vi "TempVol._activity3.vi"() -> (0 "Volume":dbl(slide) scale=0.0..1000.0, 1 "Temp":dbl(slide) scale=0.0..100.0)   [LabVIEW 2025]
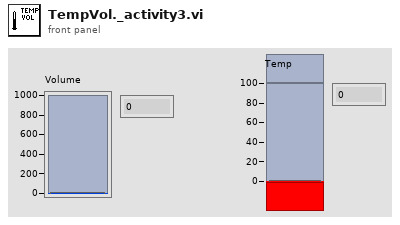
[diagram p1: front panel]
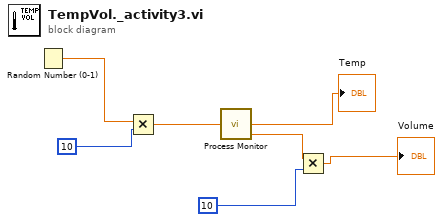
[diagram p0: block diagram]
diagram:
  n1 = Random Number (0-1)() -> (number: 0 to 1=w6:dbl)
  n2 = Multiply(x=w6, y=10) -> (x*y=w5:dbl)
  n3 = call "Process Monitor.vi"("Index"=w5) -> ("Temperature"=→"Temp":dbl, "Volume"=w3:dbl)  [unwired: 1 out]
  n4 = Multiply(x=w3, y=10) -> (x*y=→"Volume":dbl)
